vi "Simple-Waveform.vi"() -> ()   [LabVIEW 2014]
uses:
  <vilib>/measure/NI_MABase.lvlib
panel:
  in  "signal type":T1(ring)
  in  "phase":dbl format="%.2p"
  in  "frequency":dbl=10.0 format="%0.2p"
  in  "amplitude":dbl=1.0 format="%0.2p"
  in  "stop":bool
  out "Waveform Graph":waveform(dbl)(graph)
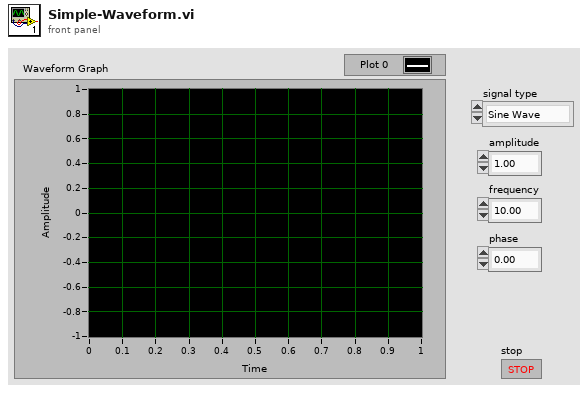
[diagram p1: front panel]
types:
  T1 = enum16{"Sine Wave", "Triangle Wave", "Square Wave", "Sawtooth Wave"}
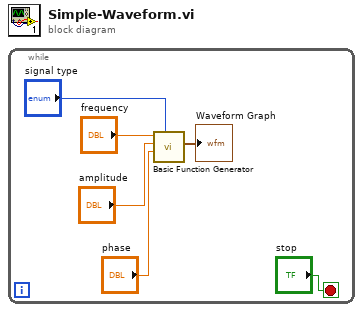
[diagram p0: block diagram]
diagram:
  n1 = while {
    stop <- "stop" stop-if-true
    n2 = call <vilib>:"Basic Function Generator.vi"("signal type"="signal type", "phase"="phase", "amplitude"="amplitude", "frequency"="frequency") -> ("signal out"=→"Waveform Graph":waveform(dbl))  [unwired: 5 in, 2 out]
  }
